vi "Create plots.vi"(6 "Relative time":bool, 7 "Data reduction":T1={"Clip time"=FALSE, "Tiime 0"=0.0, "Time 1"=0.0, "Maximum data points"=1, "Decimation method"=enum."Min-Max"}, 8 "error in (no error)":errorcluster, 11 "Data record":T2={"File path"=path "", "Channels"=[], "Group"="Untitled"}) -> (0 "error out":errorcluster, 1 "Y names":string[](array[string]), 2 "Plots":cluster{dbl[], dbl[]}[](array[cluster]) {"?" format="%#_10g"}, 3 "Data record out":T2={"File path"=path "", "Channels"=[], "Group"="Untitled"}, 4 "X-axis name":string)   [LabVIEW 2021]
uses:
  Controls/Data Viewer Entry.ctl
  Controls/Channel name entry.ctl
  Controls/Data reduction.ctl
  dc840fb0-f6f7-5a43-b4fd-bdeb8ee518a3.vi
  19a15fa6-5558-dc4d-9c97-a9e68acb042a.vi
  a998a4e5-2418-be46-9a70-433a6a432b61.vi
  dc840fb0-f6f7-5a43-b4fd-bdeb8ee518a3.vi/49e7188e-2f58-459d-91c6-4f4d8fd6d4d0.vi
  19a15fa6-5558-dc4d-9c97-a9e68acb042a.vi/49e7188e-2f58-459d-91c6-4f4d8fd6d4d0.vi
  a998a4e5-2418-be46-9a70-433a6a432b61.vi/49e7188e-2f58-459d-91c6-4f4d8fd6d4d0.vi
  Get TDMS channel info.vi
  <vilib>/measure/maresamp.llb/Resample Waveforms (single shot).vi
  <vilib>/measure/maresamp.llb/Resample Waveform (single shot).vi
  Utilities/Waveform/AvrgDecimate.vi
  Utilities/Waveform/MaxMinDecimate.vi
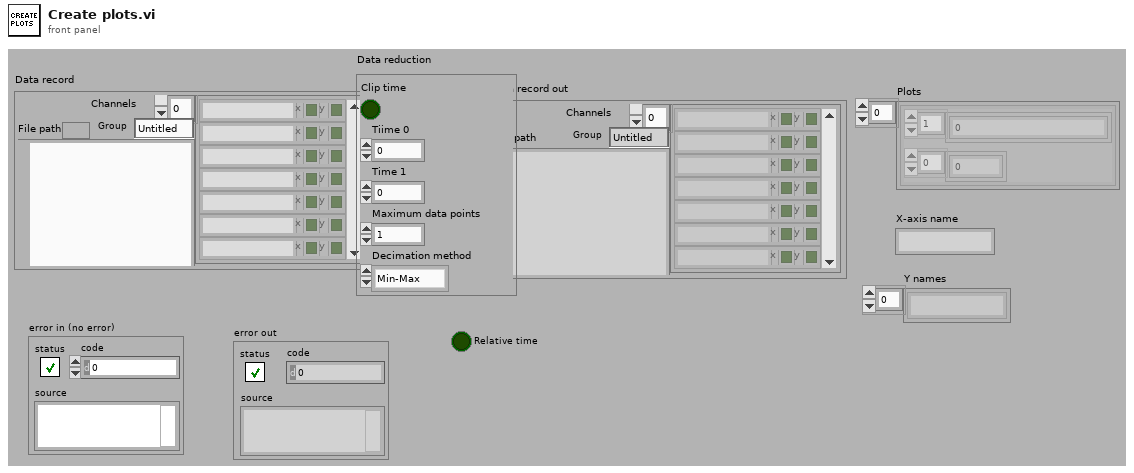
[diagram p1: front panel]
types:
  T1 = typedef "Data reduction.ctl" = cluster{"Clip time":bool, "Tiime 0":dbl, "Time 1":dbl, "Maximum data points":i32, "Decimation method":enum16{"coerce", "linear", "spline", "Min-Max", "Average"}}
  T2 = typedef "Data Viewer Entry.ctl" = cluster{"File path":path, "Channels":T3[], "Group":string}
  T3 = typedef "Channel name entry.ctl" = cluster{"Name":string, "x":bool, "y":bool}
  T4 = enum16{"open", "open or create", "create or replace", "create", "open (read-only)"}
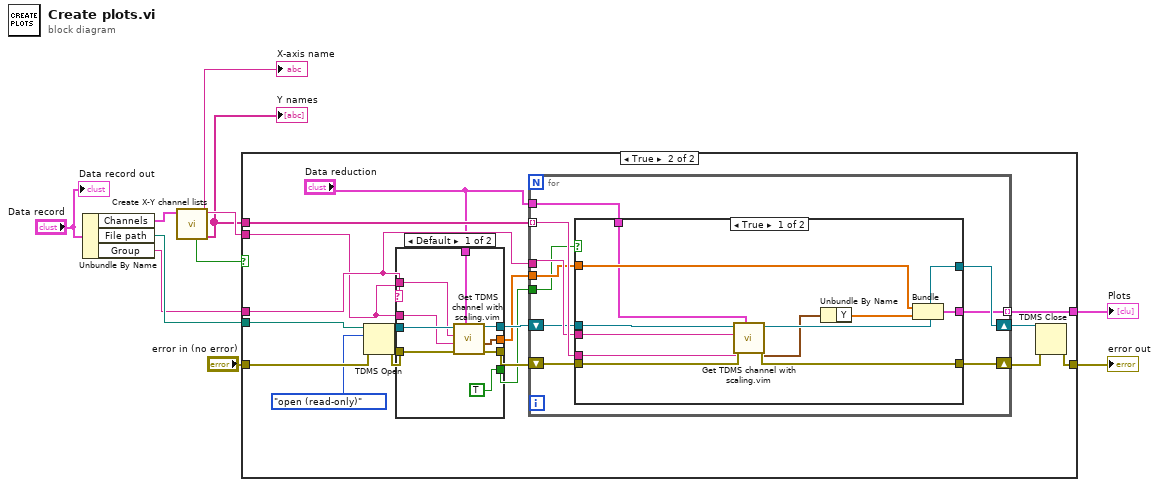
[diagram p0: block diagram]
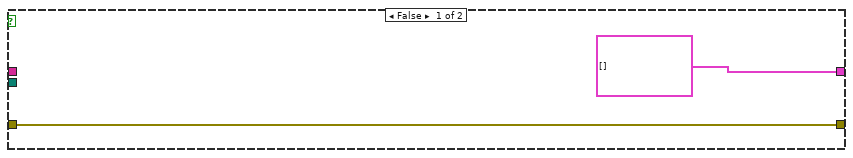
[diagram p2: hidden frame]
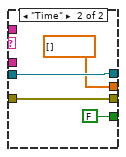
[diagram p3: hidden frame]
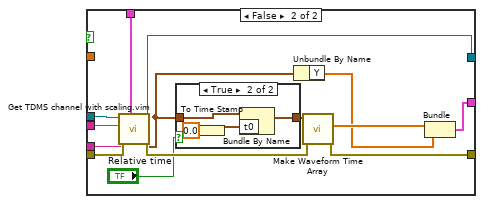
[diagram p4: hidden frame]
diagram:
  n1 = Unbundle By Name("Data record") -> ("Channels"=w8:T3[], "File path"=w10:path, "Group"=w1:string)
  n2 = call "Create X-Y channel lists.vi"("Channels to plot"=w8) -> ("Y names"=w3:string[], "X-axis name"=w5:string, "Plots exist"=w2:bool)  [unwired: 6 in, 2 out]
  "Y names" <- w3
  "X-axis name" <- w5
  n3 = case shown="True" w2 {
    tunnel: w10 -> [_ w28]
    tunnel: "error in (no error)" -> [w12 w27]
    tunnel: w3 -> [_ w24]
    tunnel: w1 -> [_ w23]
    tunnel: [cluster{dbl[], "Y":dbl[]}[] [] w20] -> w7
    tunnel: w5 -> [_ w19]
    tunnel: [w12 w14] -> w4
    frame False {
    }
    frame True {
      n4 = TDMS Open(8:w27, 10:T4."open (read-only)" ("operation (0:open)"), 11:w28) -> (0:w29:errorcluster, 3:w25:refnum<k34>)  [unwired: 4 in]
      n5 = case shown="Default" w19 {
        tunnel: w29 -> [w38 w42]
        tunnel: [w37 w42] -> w26
        tunnel: w25 -> [w36 w41]
        tunnel: w19 -> [w35 _]
        tunnel: w23 -> [w34 _]
        tunnel: [w33 w41] -> w22
        tunnel: [w32 dbl[] []] -> w21
        tunnel: [TRUE FALSE] -> w18
        tunnel: "Data reduction" -> [w30 _]
        frame Default {
          n6 = call "Get TDMS channel with scaling.vim"("Clip/desimate"=w30, "Error In"=w38, "Channel name"=w35, "group name"=w34, "tdms file"=w36) -> ("Error Out"=w37:errorcluster, "output waveform"=w32:waveform(sgl), "tdms file out"=w33:refnum<k34>)  [unwired: 4 in]
        }
        frame "Time" {
        }
      }
      n7 = for {
        tunnel: w24 -> [w51] mode=indexing
        tunnel: w23 -> [w50]
        shift-right: [w48] -> w13
        shift-left: w22 -> [w49]
        shift-right: [w47] -> w17
        shift-left: w26 -> [w52]
        tunnel: w21 -> [w46]
        tunnel: [w45] -> w20 mode=indexing
        tunnel: w18 -> [w44]
        tunnel: "Data reduction" -> [w43]
        n8 = case shown="True" w44 {
          tunnel: w52 -> [w61 w74]
          tunnel: w51 -> [w56 w71]
          tunnel: w50 -> [w55 w72]
          tunnel: w49 -> [w59 w73]
          tunnel: [w58 w70] -> w48
          tunnel: [w60 w76] -> w47
          tunnel: w46 -> [w63 _]
          tunnel: [w62 w77] -> w45
          tunnel: w43 -> [w53 w68]
          frame True {
            n9 = call "Get TDMS channel with scaling.vim"("Clip/desimate"=w53, "Error In"=w61, "Channel name"=w56, "group name"=w55, "tdms file"=w59) -> ("Error Out"=w60:errorcluster, "output waveform"=w57:waveform(sgl), "tdms file out"=w58:refnum<k34>)  [unwired: 4 in]
            n10 = Unbundle By Name(w57) -> ("Y"=w54:sgl[])
            n11 = Bundle(w63, "Y"=w54) -> (w62:cluster{dbl[], "Y":sgl[]})  [unwired: 1 out]
          }
          frame False {
            n12 = call "Get TDMS channel with scaling.vim"("Clip/desimate"=w68, "Error In"=w74, "Channel name"=w71, "group name"=w72, "tdms file"=w73) -> ("Error Out"=w69:errorcluster, "output waveform"=w66:waveform(sgl), "tdms file out"=w70:refnum<k34>)  [unwired: 4 in]
            n13 = case shown="True" "Relative time" {
              tunnel: w66 -> [w78 w82]
              tunnel: [w78 w81] -> w65
              frame False {
              }
              frame True {
                n14 = To Time Stamp(1:0.0) -> (0:w79:timestamp)
                n15 = Bundle By Name(cluster=w82, "t0"=w79) -> (w81:waveform(sgl))
              }
            }
            n16 = Unbundle By Name(w66) -> ("Y"=w67:sgl[])
            n17 = call "Make Waveform Time Array.vi"("error in (no error)"=w69, "waveform in"=w65) -> ("error out"=w76:errorcluster, "X array"=w75:dbl[])  [unwired: 8 in]
            n18 = Bundle("X array"=w75, "Y"=w67) -> (w77:cluster{"X array":dbl[], "Y":sgl[]})  [unwired: 1 out]
          }
        }
      }
      n19 = TDMS Close(8:w17, 11:w13) -> (0:w14:errorcluster)  [unwired: 1 out]
    }
  }
  "error out" <- w4
  "Plots" <- w7
  "Data record out" <- "Data record"
